vi "example_GArrayDownload.vi"() -> ()   [LabVIEW 2020]
uses:
  <vilib>/Galil/resources/gclib32/gclib32.lvlib
panel:
  out "Response":string
  in  "Command":string="DM A[100]"
  out "Response 2":string=" \r\n:"
  in  "Command 2":string="MG A[0]"
  out "Error Out":errorcluster
  in  "IP Address":string="192.168.1.77"
  in  "Array Elements":string="100,120,140,160,180,200"
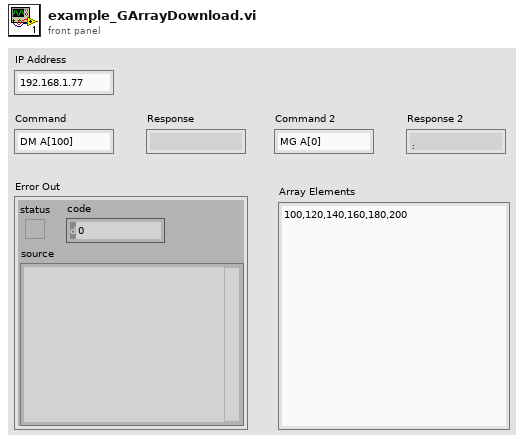
[diagram p1: front panel]
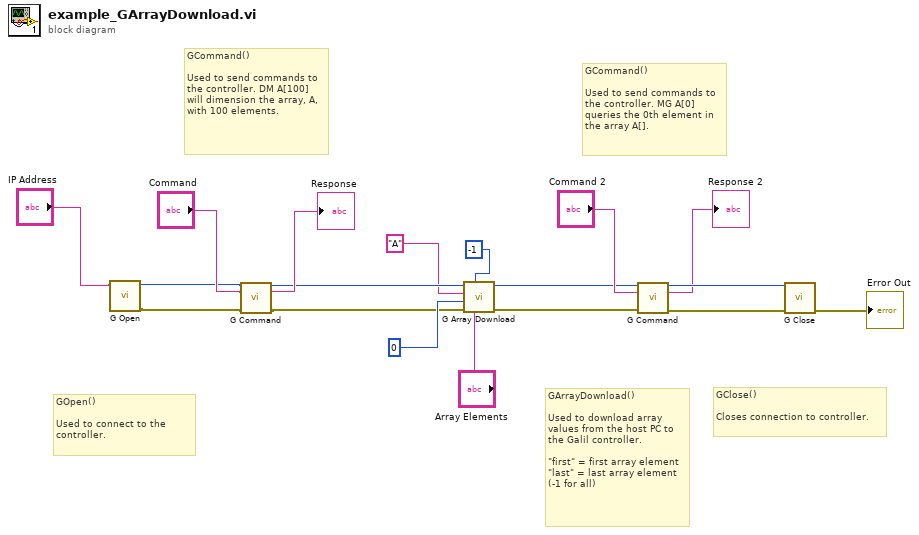
[diagram p0: block diagram]
diagram:
  # "GCommand()\n\nUsed to send commands to the controller. MG A[0] queries the 0th element in the array A[]."
  # "GClose()\n\nCloses connection to controller."
  # "GCommand()\n\nUsed to send commands to the controller. DM A[100] will dimension the array, A, with 100 elements."
  # "GOpen()\n\nUsed to connect to the controller."
  # "GArrayDownload()\n\nUsed to download array values from the host PC to the Galil controller.\n\n\"first\" = first array element\n\"last\" = last array element (-1 for all)"
  n1 = call <vilib>:"G Open.vi"("address"="IP Address") -> ("error out"=w16:errorcluster, "g out"=w11:u32)  [unwired: 8 in]
  n2 = call <vilib>:"G Command.vi"("g"=w11, "command"="Command", "error in (no error)"=w16) -> ("g out"=w7:u32, "buffer out"=→"Response":string, "error out"=w4:errorcluster)  [unwired: 10 in]
  n3 = call <vilib>:"G Array Download.vi"("buffer"="Array Elements", "last"=-1, "error in (no error)"=w4, "first"=0, "array_name"="A", "g"=w7) -> ("error out"=w3:errorcluster, "g out"=w2:u32)  [unwired: 4 in]
  n4 = call <vilib>:"G Command.vi"("g"=w2, "command"="Command 2", "error in (no error)"=w3) -> ("g out"=w14:u32, "buffer out"=→"Response 2":string, "error out"=w15:errorcluster)  [unwired: 10 in]
  n5 = call <vilib>:"G Close.vi"("error in (no error)"=w15, "g"=w14) -> ("error out"=→"Error Out":errorcluster)  [unwired: 9 in]
